vi "Record.vi"() -> ()   [LabVIEW 2013, in "Phonocardiography.lvlib"]
uses:
  Phonocardiography.lvlib
  <vilib>/sound2/lvsound2.llb/Sampling Mode.ctl
  <vilib>/sound2/lvsound2.llb/Sound Data Format.ctl
  <vilib>/sound2/lvsound2.llb/Sound Input Read (DBL).vi
panel:
  in  "Save to":path
  in  "Samples per\nLoop":i32=8192
  in  "Device ID":u32
  out "Heart sound":waveform(dbl)(graph)
  in  "Stop & Save":bool
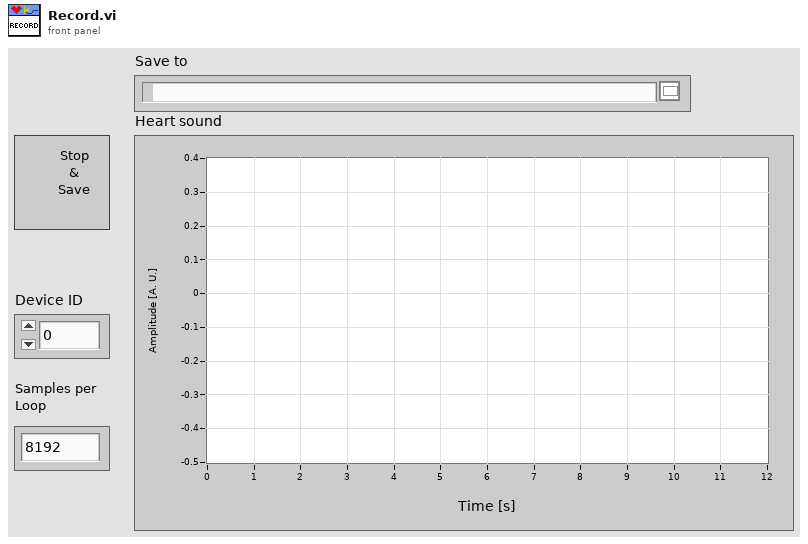
[diagram p1: front panel]
types:
  T1 = typedef "Sound Data Format.ctl" = cluster{"sample rate (S/s)":dbl, "number of channels":i32, "bits per sample":i32}
  T2 = typedef "Sampling Mode.ctl" = i32
  T3 = typedef "Sound Input Task ID.ctl" = u32
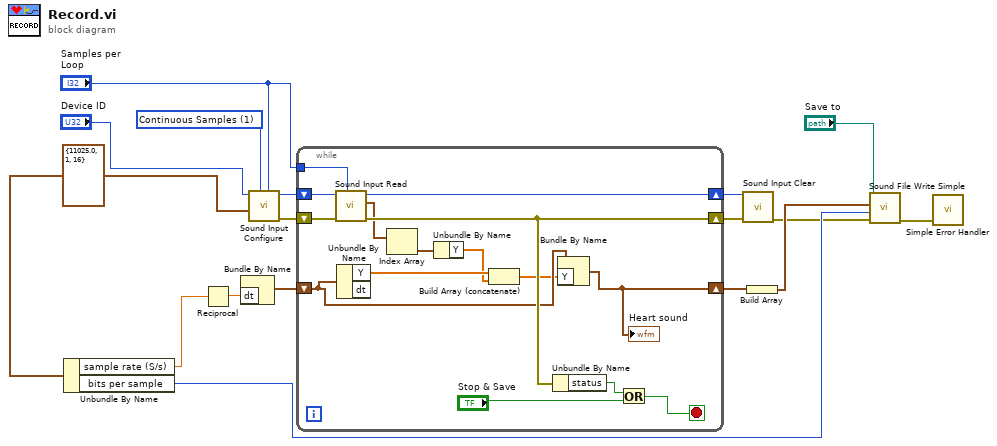
[diagram p0: block diagram]
diagram:
  w10 = T1 {"sample rate (S/s)"=11025.0, "number of channels"=1, "bits per sample"=16} ("Sound Format")
  w17 = T2 1 items=["Finite Samples", "Continuous Samples"] ("sample mode")
  n1 = Unbundle By Name(w10) -> ("sample rate (S/s)"=w4:dbl, "bits per sample"=w8:i32)
  n2 = Reciprocal(x=w4) -> (1/x=w6:dbl)
  n3 = Bundle By Name("dt"=w6) -> (w5:waveform(dbl))  [unwired: 1 in]
  n4 = call <vilib>:"Sound Input Configure.vi"("number of samples/ch"="Samples per\nLoop", "sample mode"=w17, "sound format"=w10, "device ID"="Device ID") -> ("error out"=w13:errorcluster, "task ID"=w14:T3)  [unwired: 6 in]
  n5 = while {
    tunnel: "Samples per\nLoop" -> [w29]
    shift-right: [w30] -> w15
    shift-left: w14 -> [w31]
    shift-right: [w27] -> w16
    shift-left: w13 -> [w32]
    shift-right: [w20] -> w7
    shift-left: w5 -> [w22]
    stop <- w28 stop-if-true
    n6 = call-poly <vilib>:"Sound Input Read.vi"("number of samples/ch"=w29, "error in (no error)"=w32, "task ID"=w31) -> ("error out"=w27:errorcluster, "data"=w26:waveform(dbl)[], "task ID out"=w30:T3)  [unwired: 6 in]
    n7 = Unbundle By Name(w22) -> ("Y"=w24:dbl[])  [unwired: 1 out]
    n8 = Index Array(array=w26) -> (element=w25:waveform(dbl))  [unwired: 1 in]
    n9 = Unbundle By Name(w25) -> ("Y"=w23:dbl[])
    n10 = Build Array (concatenate)(w24, w23) -> (w21:dbl[])
    n11 = Unbundle By Name(w27) -> ("status"=w19:bool)
    n12 = Bundle By Name(cluster=w22, "Y"=w21) -> (w20:waveform(dbl))
    "Heart sound" <- w20
    n13 = Or(x=w19, y="Stop & Save") -> (x .or. y?=w28:bool)
  }
  n14 = call <vilib>:"Sound Input Clear.vi"("error in (no error)"=w16, "task ID"=w15) -> ("error out"=w1:errorcluster)  [unwired: 9 in]
  n15 = Build Array(w7) -> (w9:waveform(dbl)[])
  n16 = call <vilib>:"Sound File Write Simple.vi"("error in (no error)"=w1, "bits per sample"=w8, "data"=w9, "path"="Save to") -> ("error out"=w3:errorcluster)  [unwired: 6 in, 1 out]
  n17 = call <vilib>:"Simple Error Handler.vi"("error in (no error)"=w3) -> ()  [unwired: 4 in, 5 out]
